vi "niRFUtil RFHS Benchmark Mgr.vi"(0 "String":string, 2 "What":enum16{"Register", "Get Tree", "Reset Database"}(ring), 5 "Owner":i32) -> (4 "ID":u32, 6 "Tree":T1[](array[typedef]))   [LabVIEW 2015, in "niRFUtil.lvlib"]
uses:
  niRFUtil.lvlib
  niRFUtil RFHS Benchmark TaskMgrInfo.ctl
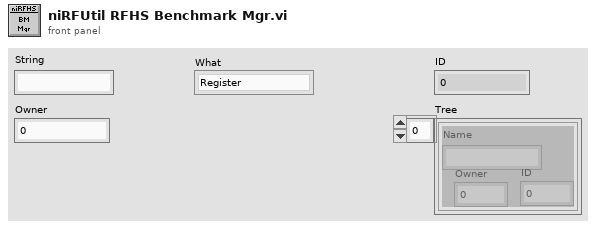
[diagram p1: front panel]
types:
  T1 = typedef "niRFUtil.lvlib/niRFUtil RFHS Benchmark TaskMgrInfo.ctl" = cluster{"Name":string, "Owner":i32, "ID":i32}
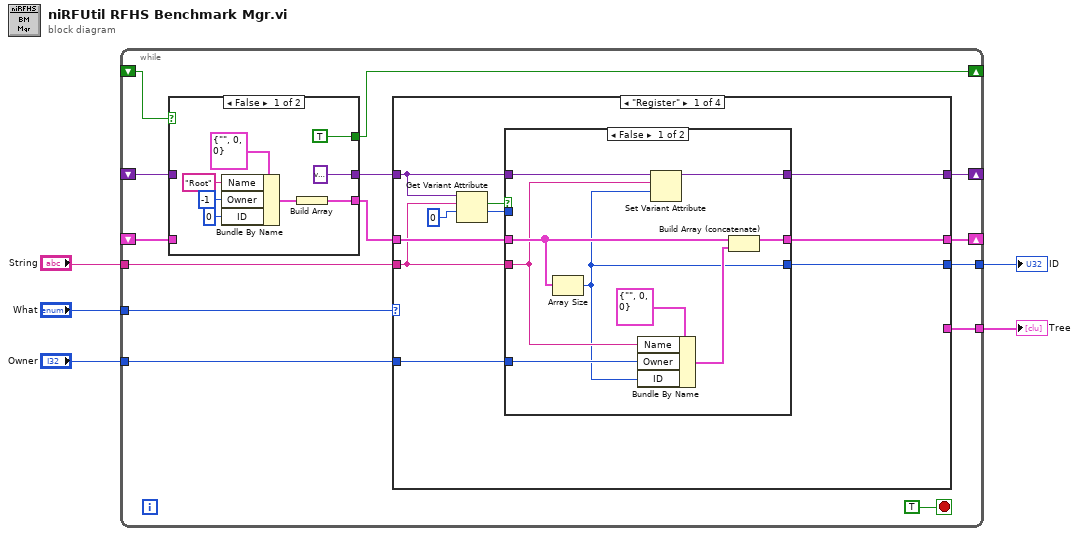
[diagram p0: block diagram]
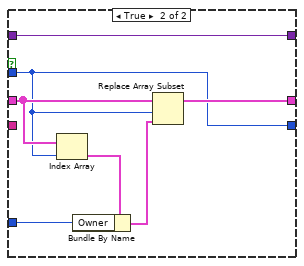
[diagram p3: hidden frame]
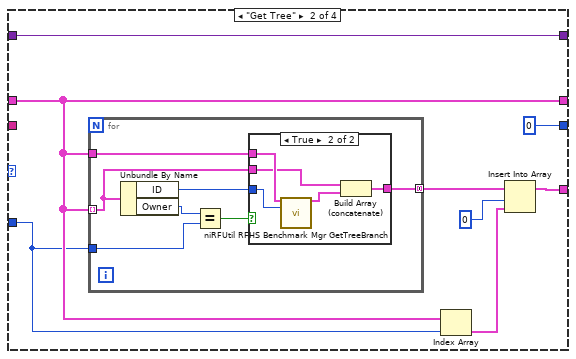
[diagram p4: hidden frame]
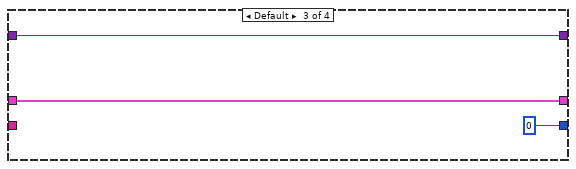
[diagram p6: hidden frame]
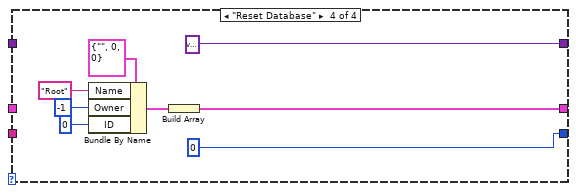
[diagram p7: hidden frame]
diagram:
  n1 = while {
    shift-right: [w16] -> _
    shift-left: _ -> [w12]
    tunnel: "What" -> [w19]
    tunnel: "String" -> [w18]
    shift-right: [w15] -> _
    shift-left: _ -> [w10]
    tunnel: [w17] -> w2
    shift-right: [w13] -> _
    shift-left: _ -> [w14]
    tunnel: "Owner" -> [w8]
    tunnel: [w7] -> w1
    stop <- TRUE stop-if-true
    n2 = case shown="False" w14 {
      selector: w14 -> [_ w30]
      tunnel: [TRUE w30] -> w13
      tunnel: w12 -> [_ w29]
      tunnel: [variant w29] -> w11
      tunnel: w10 -> [_ w28]
      tunnel: [w23 w28] -> w9
      frame False {
        n3 = Bundle By Name(cluster=T1 {"Name"="", "Owner"=0, "ID"=0} ("Data"), "Name"="Root", "Owner"=-1, "ID"=0) -> (w24:T1)
        n4 = Build Array(w24) -> (w23:T1[])
      }
      frame True {
      }
    }
    n5 = case shown="\"Register\"" w19 {
      tunnel: w11 -> [w39 w64 w78 _]
      tunnel: w18 -> [w33 _ _ _]
      tunnel: w9 -> [w36 w60 w79 _]
      tunnel: [w35 0 0 0] -> w17
      tunnel: [w34 w64 w78 variant] -> w16
      tunnel: [w32 w60 w79 w81] -> w15
      tunnel: w8 -> [w31 w59 _ _]
      tunnel: [_ w62 _ _] -> w7
      frame "Register" {
        n6 = Get Variant Attribute(Variant=w39, name=w33, default value (empty Variant)=0) -> (found=w40:bool, value=w37:i32)  [unwired: 1 in, 2 out]
        n7 = case shown="False" w40 {
          tunnel: w39 -> [w49 w56]
          tunnel: w37 -> [_ w51]
          tunnel: w36 -> [w47 w55]
          tunnel: [w41 w51] -> w35
          tunnel: [w48 w56] -> w34
          tunnel: w33 -> [w45 _]
          tunnel: [w46 w52] -> w32
          tunnel: w31 -> [w44 w53]
          frame False {
            n8 = Array Size(array=w47) -> (size(s)=w41:i32)
            n9 = Bundle By Name(cluster=T1 {"Name"="", "Owner"=0, "ID"=0} ("Data"), "Name"=w45, "Owner"=w44, "ID"=w41) -> (w43:T1)
            n10 = Set Variant Attribute(Variant=w49, name=w45, value=w41) -> (Variant out=w48:variant)  [unwired: 1 in, 2 out]
            n11 = Build Array (concatenate)(w47, w43) -> (w46:T1[])
          }
          frame True {
            n12 = Index Array(array=w55, index=w51) -> (element=w54:T1)
            n13 = Bundle By Name(cluster=w54, "Owner"=w53) -> (w50:T1)
            n14 = Replace Array Subset(array=w55, new element=w50, index=w51) -> (w52:T1[])
          }
        }
      }
      frame "Get Tree" {
        n15 = for {
          tunnel: w60 -> [w65] mode=indexing
          tunnel: w59 -> [w70]
          tunnel: w60 -> [w69]
          tunnel: [w68] -> w61 mode=concatenating
          n16 = Unbundle By Name(w65) -> ("ID"=w66:i32, "Owner"=w71:i32)
          n17 = Equal?(x=w71, y=w70) -> (x = y?=w67:bool)
          n18 = case shown="True" w67 {
            tunnel: w69 -> [_ w76]
            tunnel: [_ w73] -> w68
            tunnel: w66 -> [_ w74]
            tunnel: w65 -> [_ w72]
            frame False {
            }
            frame True {
              n19 = call "niRFUtil RFHS Benchmark Mgr GetTreeBranch.vi"("Tree"=w76, "Owner"=w74) -> ("Branch"=w75:T1[])  [unwired: 13 in]
              n20 = Build Array (concatenate)(w72, w75) -> (w73:T1[])
            }
          }
        }
        n21 = Index Array(array=w60, index=w59) -> (element=w58:T1)
        n22 = Insert Into Array(array=w61, index=0, new element=w58) -> (w62:T1[])
      }
      frame Default {
      }
      frame "Reset Database" {
        n23 = Bundle By Name(cluster=T1 {"Name"="", "Owner"=0, "ID"=0} ("Data"), "Name"="Root", "Owner"=-1, "ID"=0) -> (w84:T1)
        n24 = Build Array(w84) -> (w81:T1[])
      }
    }
  }
  "ID" <- w2
  "Tree" <- w1
